vi "Toggle Power.vi"(8 "error in (no error)":errorcluster, 10 "Power On?":bool, 11 "TCP 380 in":refnum<class "TCP 380.lvclass">) -> (0 "error out":errorcluster, 3 "TCP 380 out":refnum<class "TCP 380.lvclass">)   [LabVIEW 2021, in "TCP 380.lvclass"]
uses:
  TCP 380.lvclass
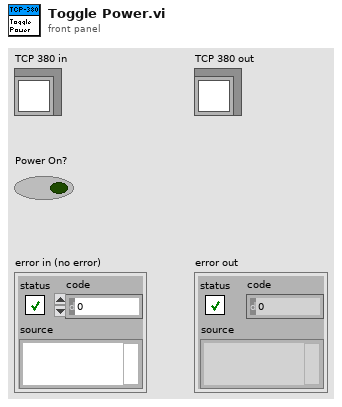
[diagram p1: front panel]
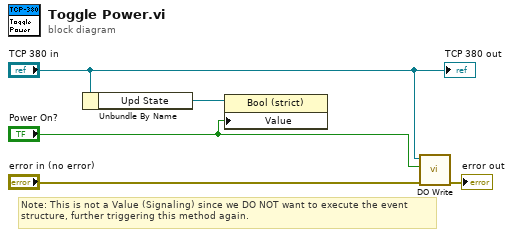
[diagram p0: block diagram]
diagram:
  # "Note: This is not a Value (Signaling) since we DO NOT want to execute the event structure, further triggering this method again."
  n1 = Unbundle By Name("TCP 380 in") -> ("Upd State"=w2:refnum<vi>)
  n2 = property class="Bool (strict)"(reference=w2, "Value"="Power On?") -> ()  [unwired: 1 in, 2 out]
  n3 = call "DO Write.vi"("error in (no error)"="error in (no error)", "Digital Output"="Power On?", "TCP 380 in"="TCP 380 in") -> ("error out"=→"error out":errorcluster)  [unwired: 8 in]
  "TCP 380 out" <- "TCP 380 in"
